vi "Set package_templatemessage.vi"(7 "Complete Call (T)":bool=TRUE, 8 "error in (no error)":errorcluster, 10 "package_templatemessage":T1, 11 "gRPCid":T2) -> (0 "error out":errorcluster)   [LabVIEW 2024, in "Service Template.lvlib"]
uses:
  Service Template.lvlib
  gRPC lv Support/grpc-lvsupport/grpc-lvsupport.lvlib
  dcc74a39-081a-4bdd-860b-8ed792803c96.vi
  package_templatemessage.ctl
  c8cd2a7d-3f0e-47f4-bd6c-d8bf1e02ce4e.vi
  gRPC lv Support/grpc-lvsupport/grpcId.ctl
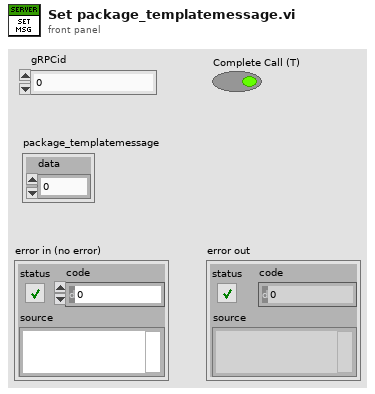
[diagram p1: front panel]
types:
  T1 = typedef "Service Template.lvlib/package_templatemessage.ctl" = cluster{"data":sgl}
  T2 = typedef "grpc-lvsupport.lvlib/grpcId.ctl" = u64
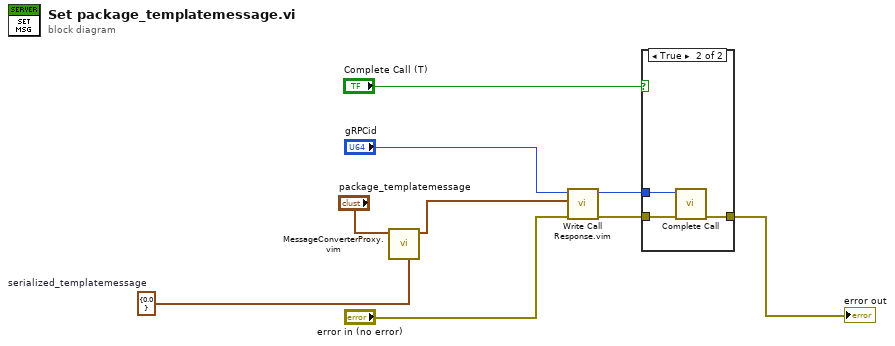
[diagram p0: block diagram]
diagram:
  w2 = T1 {"data"=0.0}  # serialized_templatemessage
  n1 = call "MessageConverterProxy.vim"("package_templatemessage_type"=w2, "example_SignalParameters_Data"="package_templatemessage") -> ("package_templatemessage"=w1:T1)  [unwired: 9 in]
  n2 = call "Write Call Response.vim"("error in"="error in (no error)", "Response Data"=w1, "gRPCid in"="gRPCid") -> ("error out"=w6:errorcluster, "gRPCid out"=w7:T2)  [unwired: 7 in]
  n3 = case shown="True" "Complete Call (T)" {
    tunnel: [w10 w13] -> w9
    tunnel: w7 -> [_ w12]
    tunnel: w6 -> [w10 w11]
    frame False {
    }
    frame True {
      n4 = call "Complete Call.vi"("gRPCid"=w12, "error in"=w11) -> ("error out"=w13:errorcluster)  [unwired: 8 in]
    }
  }
  "error out" <- w9
